vi "Event Ctr, Programmable Edge.vi"() -> ()   [LabVIEW 2015]
doc: "This VI contains an event counter that increments on the hardware selected edge of the input signal. To reset the value of the counter, push the reset button.\n\nThe trigger of the event counter is set to PB1, reset to PB2, and the edge selector to SWITCH1 on the sbRIO evaluation board. The value of SWITCH1 at the start of the VI decides which edge to count on the input. This edge type will be displayed on the Edge Type indicator."
uses:
  <vilib>/Platform/TimedLoop/XDataNode/timing_clust.ctl
  <vilib>/Platform/TimedLoop/XDataNode/nitl_modes.ctl
  <vilib>/Platform/TimedLoop/XDataNode/wakeup.ctl
  <vilib>/rvi/eio/common/nirviEmuTemplateMethod_errors.vi
  <vilib>/rvi/Emulation/niFpgaSctlEmulationGetInTimedLoop.vi
  <vilib>/rvi/Emulation/niFpgaEmulationReportErrorSimple.vi
  <vilib>/rvi/Emulation/niFpgaGetClockAttributes.vi
  <vilib>/rvi/Emulation/niFpgaCriticalErrorInLSC.vi
  <vilib>/Platform/TimedLoop/XDataNode/XDataNode.xnode
  <vilib>/eio/EIONode/EIONode.xnode
  <vilib>/Platform/TimedLoop/XDataNode/XDNodeRunTimeDep.lvlib
panel:
  out "Edge Type":u8
  in  "stop":bool
  out "8-bit count":u8
  # "This VI contains an event counter that increments on the hardware selected edge of the input signal.  To reset the value of the counter, push the reset button.\n\nThe trigger of the event counter is set to PB1, reset to PB2, and the edge selector to PB1 on the LabVIEW RIO evaluation board.  The value of PB1 at the start of the VI decides which edge to count on the input, which is naturally false because the push buttons response is a small pulse from false to true and back to false. This edge type will be displayed on the Edge Type indicator, which by default is falling edge."
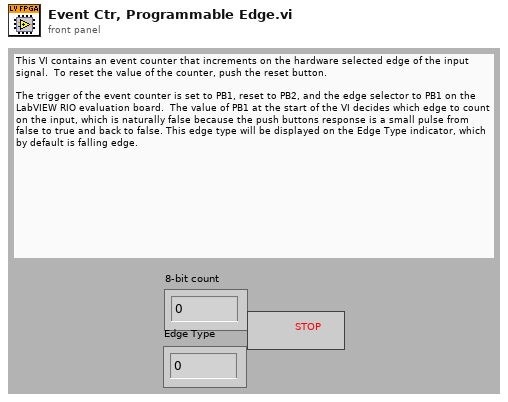
[diagram p1: front panel]
types:
  T1 = typedef "XDNodeRunTimeDep.lvlib/timing_clust.ctl" = cluster{"Expected End [f-1]":u64, "Actual End [f-1]":u64, "Finished Late? [f-1]":bool, "Expected End [i-1]":u64, "Actual End [i-1]":u64, "Finished Late? [i-1]":bool, "Expected Start [i]":u64, "Actual Start [i]":u64, "Expected Start [f]":u64, "Actual Start [f]":u64, "Source Name":string, "Structure Name":string, "Period":i64, "Deadline":i64, "Offset":i64, "Start":i64, "Priority":i32, "Timeout":i32, "Mode":T2, "Wakeup Reason":T3, "Error":errorcluster, "Source Type":string, "Secondary Source Type":string, "Global End Time":u64, "Global Start Time":u64, "Frame Duration":u64, "Iteration Duration":u64, "Assigned CPU":i32, "I/O Scan Engine Mode":u32}
  T2 = typedef "XDNodeRunTimeDep.lvlib/nitl_modes.ctl" = enum32{"No Change", "Process missed periods, maintain original phase", "Discard missed periods, maintain original phase", "Process missed periods, ignore original phase", "Discard missed periods, ignore original phase"}
  T3 = typedef "XDNodeRunTimeDep.lvlib/wakeup.ctl" = enum32{"Normal", "Aborted", "Asynchronous wakeup", "Timing source error", "Timed loop error", "Timeout"}
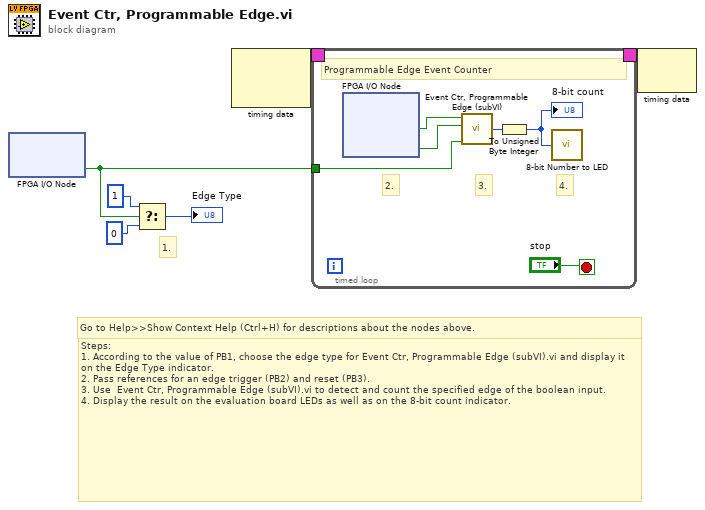
[diagram p0: block diagram]
diagram:
  # "Go to Help>>Show Context Help (Ctrl+H) for descriptions about the nodes above."
  # "1."
  # "Steps:\n1. According to the value of PB1, choose the edge type for Event Ctr, Programmable Edge (subVI).vi and display it on the Edge Type indicator. \n2. Pass references for an edge trigger (PB2) and reset (PB3).\n3. Use  Event Ctr, Programmable Edge (subVI).vi to detect and count the specified edge of the boolean input.\n4. Display the result on the evaluation board LEDs as well as on the 8-bit count indicator."
  n1 = xnode "FPGA I/O Node"() -> ("PB1"=w1:bool)  [unwired: 1 in, 1 out]
  n2 = Select(t=u8 1, s=w1, f=u8 0) -> (s? t:f=→"Edge Type":u8)
  n3 = node-c288() -> (w5:T1)  [unwired: 2 out]
  n4 = timed-loop {
    timing-out: [_] -> w6
    timing: w5 -> [_]
    tunnel: w1 -> [w9]
    stop <- "stop" stop-if-true
    # "4."
    # "3."
    # "2."
    # "Programmable Edge Event Counter"
    n5 = xnode "FPGA I/O Node"() -> ("PB1"=w7:bool, "PB2"=w8:bool)  [unwired: 2 in, 2 out]
    n6 = call "Event Ctr, Programmable Edge (subVI).vi"("Edge Type (false)"=w9, "Reset"=w8, "Edge Trigger"=w7) -> ("16 bit Count"=w11:u16)  [unwired: 1 out]
    n7 = To Unsigned Byte Integer(number=w11) -> (unsigned 8bit integer=w10:u8)
    "8-bit count" <- w10
    n8 = call "8-bit Number to LED.vi"("6-bit Unsigned\n Number (0-63)"=w10) -> ()  [unwired: 1 out]
  }
  n9 = node-c288(w6) -> ()  [unwired: 1 out]
